vi "Cargo Align.vi"() -> (2 "Wheel":dbl=-0.027675343784815974, 3 "Throttle":dbl=-0.0261269211769104)   [LabVIEW 2020]
uses:
  <vilib>/Rock Robotics/Network Tables/NT Read Number.vi
  <vilib>/addons/control/pid/pid.llb/PID (DBL).vi
  <vilib>/addons/control/pid/NI_PID_pid.lvlib
panel:
  in  "OutputRange":cluster{"output high":dbl, "output low":dbl}={"output high"=1.0, "output low"=-1.0} {"output low" format="%.2f"; "output high" format="%.2f"}
  in  "ThrottlePID":T1={"proportional gain (Kc)"=0.018, "integral time (Ti, min)"=0.0, "derivative time (Td, min)"=0.0} {"derivative time (Td, min)" format="%.3f"; "integral time (Ti, min)" format="%.3f"; "proportional gain (Kc)" format="%.3f"}
  in  "WheelPID":T1={"proportional gain (Kc)"=0.02, "integral time (Ti, min)"=0.0, "derivative time (Td, min)"=1e-05} {"derivative time (Td, min)" format="%.3f"; "integral time (Ti, min)" format="%.3f"; "proportional gain (Kc)" format="%.3f"}
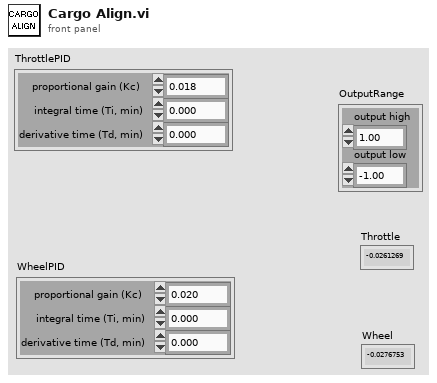
[diagram p1: front panel]
types:
  T1 = cluster{"proportional gain (Kc)":dbl, "integral time (Ti, min)":dbl, "derivative time (Td, min)":dbl}
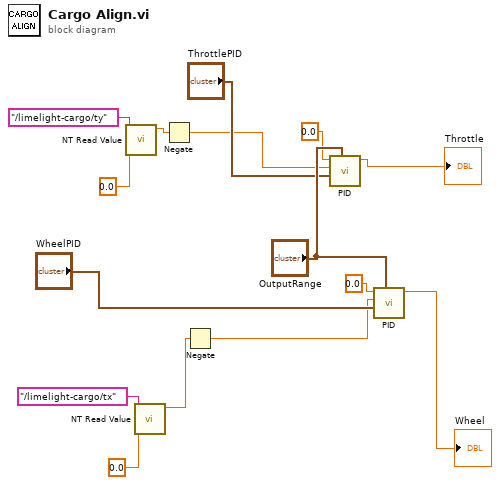
[diagram p0: block diagram]
diagram:
  n1 = call-poly <vilib>:"NT Read Value.vi"("Default Value"=0.0, "Name"="/limelight-cargo/ty") -> ("Numeric"=w3:dbl)  [unwired: 8 in, 1 out]
  n2 = call-poly <vilib>:"NT Read Value.vi"("Default Value"=0.0, "Name"="/limelight-cargo/tx") -> ("Numeric"=w8:dbl)  [unwired: 8 in, 1 out]
  n3 = Negate(x=w3) -> (-x=w2:dbl)
  n4 = Negate(x=w8) -> (-x=w1:dbl)
  n5 = call-poly <vilib>:"PID.vi"("output range"="OutputRange", "PID gains"="ThrottlePID", "process variable"=w2, "setpoint"=0.0) -> ("output"=→"Throttle":dbl)  [unwired: 6 in, 1 out]
  n6 = call-poly <vilib>:"PID.vi"("output range"="OutputRange", "PID gains"="WheelPID", "process variable"=w1, "setpoint"=0.0) -> ("output"=→"Wheel":dbl)  [unwired: 6 in, 1 out]
